vi "SimpleAAV.vi"() -> ()   [LabVIEW 2017]
panel:
  out "Average Value":dbl
  out "Waveform Graph":dynamicdata(graph)
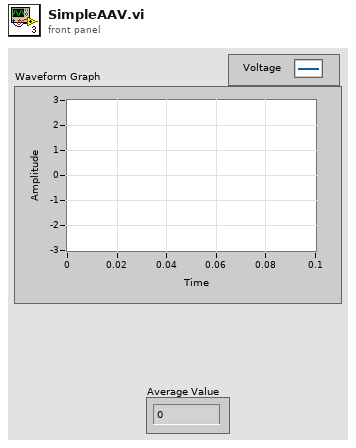
[diagram p1: front panel]
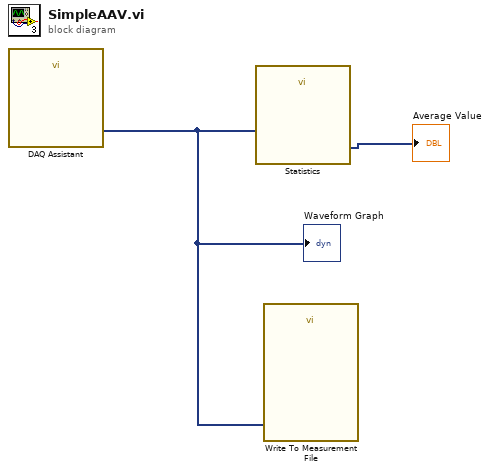
[diagram p0: block diagram]
diagram:
  n1 = call "DAQ Assistant"() -> ("data"=w1:dynamicdata)  [unwired: 17 in, 2 out]
  "Waveform Graph" <- w1
  n2 = call "Statistics"("Signals"=w1) -> ("Arithmetic Mean"=→"Average Value":dynamicdata)  [unwired: 25 in, 1 out]
  n3 = call "Write To Measurement File"("Signals"=w1) -> ()  [unwired: 16 in, 3 out]
